vi "Set forLogging.vi"(8 "error in (no error)":errorcluster, 10 "forLogging":string, 11 "niDTS Comm String in":refnum<class "niDTS Comm String.lvclass">) -> (0 "error out":errorcluster, 3 "niDTS Comm String out":refnum<class "niDTS Comm String.lvclass">)   [LabVIEW 2015, in "niDTS CommLib.lvlib" / "niDTS Comm String.lvclass"]
uses:
  niDTS Comm String.lvclass
  niDTS Comm String.lvclass/niDTS Comm String.ctl
  Framework/Logger/Includes/niDTS Logger INC Log Element Type.ctl
  Framework/Logger/Objects/BASE_class/niDTS Logger.lvclass
  Framework/niDTS Framework.lvlib
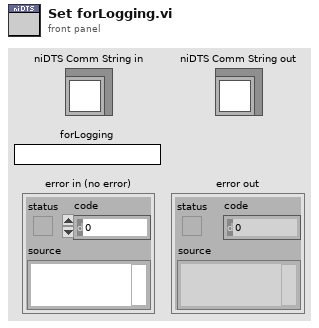
[diagram p1: front panel]
types:
  T1 = typedef "niDTS Framework.lvlib/niDTS Logger INC Log Element Type.ctl" = enum16{"Error", "Warning", "Information", "Debugging"}
  T2 = typedef "niDTS Framework.lvlib/niDTS Logger INC Handle.ctl" = refnum<data-value>
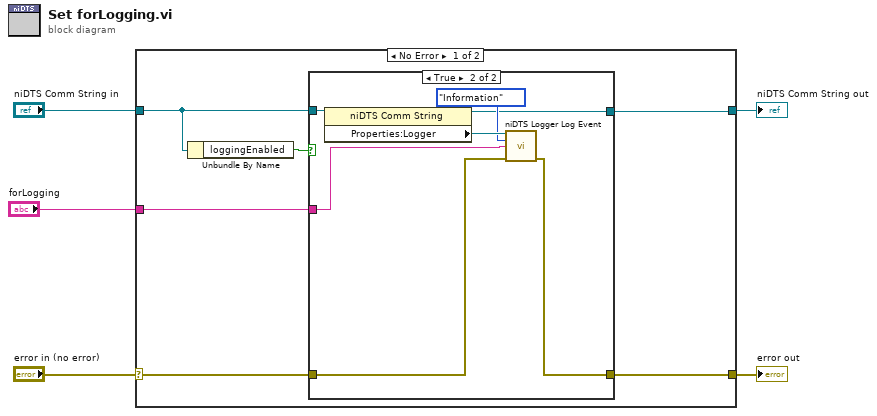
[diagram p0: block diagram]
diagram:
  n1 = case shown="No Error" "error in (no error)" {
    selector: "error in (no error)" -> [w8 w22]
    tunnel: [w7 w22] -> w4
    tunnel: [w6 w21] -> w2
    tunnel: "niDTS Comm String in" -> [w11 w21]
    tunnel: "forLogging" -> [w9 _]
    frame No Error {
      n2 = Unbundle By Name(w11) -> ("loggingEnabled"=w10:bool)
      n3 = case shown="True" w10 {
        tunnel: w11 -> [w13 w20]
        tunnel: w9 -> [_ w17]
        tunnel: w8 -> [w12 w16]
        tunnel: [w12 w15] -> w7
        tunnel: [w13 w14] -> w6
        frame False {
        }
        frame True {
          n4 = property class="niDTS Comm String"(reference=w20) -> (reference out=w14:refnum<class "niDTS Comm String.lvclass">, "Properties:Logger"=w19:T2)  [unwired: 1 in, 1 out]
          n5 = call "niDTS Logger Log Event.vi"("Logger Handle"=w19, "Type"=niDTS_Logger_INC_Log_Element_Type."Information", "Description/Data"=w17, "error in (no error)"=w16) -> ("error out"=w15:errorcluster)  [unwired: 9 in, 2 out]
        }
      }
    }
    frame Error {
    }
  }
  "error out" <- w4
  "niDTS Comm String out" <- w2
